vi "AD5781SetVolt.vi"(3 "Send":bool=TRUE, 5 "SetVolt":u32 format="%032b") -> (2 "timedOut":bool)   [LabVIEW 2014]
uses:
  <vilib>/rvi/Emulation/niFpgaGetClockAttributes.vi
  <vilib>/rvi/Emulation/niFpgaSctlEmulationGetInTimedLoop.vi
  <vilib>/rvi/Emulation/niFpgaEmulationReportErrorSimple.vi
  <vilib>/rvi/Emulation/niFpgaCriticalErrorInLSC.vi
  <vilib>/rvi/interface/RandomDataEmulation/niFpgaRandomDataHandleErrors.vi
  <vilib>/rvi/DataTransferAndStorage/Container/XNode/niFpgaContainer.xnode
  <vilib>/rvi/interface/RandomDataEmulation/nirviRandomDataFpgaReadWriteTemplate.vi
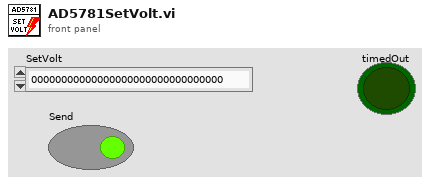
[diagram p1: front panel]
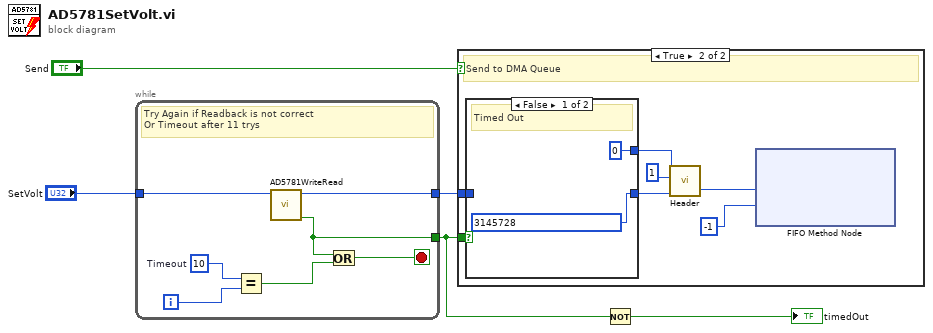
[diagram p0: block diagram]
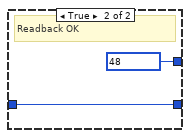
[diagram p3: hidden frame]
diagram:
  n1 = while {
    tunnel: "SetVolt" -> [w12]
    tunnel: [w7] -> w4
    tunnel: [w6] -> w3
    i -> [w11]
    stop <- w9 stop-if-true
    w10 = 10  # Timeout
    # "Try Again if Readback is not correct\nOr Timeout after 11 trys"
    n2 = Equal?(x=w10, y=w11) -> (x = y?=w8:bool)
    n3 = call "AD5781WriteRead.vi"("Write"=w12) -> ("WriteEqualsRead"=w6:bool, "Readback"=w7:u32)  [unwired: 6 in]
    n4 = Or(x=w6, y=w8) -> (x .or. y?=w9:bool)
  }
  n5 = case shown="True" "Send" {
    tunnel: w4 -> [_ w15]
    tunnel: w3 -> [_ w13]
    frame False {
    }
    frame True {
      # "Send to DMA Queue"
      n6 = case shown="False" w13 {
        tunnel: [u8 0 ("8BitHead") u8 48 ("8BitHead")] -> w19
        tunnel: w15 -> [_ w22]
        tunnel: [u32 3145728 ("Readback") w22] -> w14
        frame False {
          # "Timed Out"
        }
        frame True {
          # "Readback OK"
        }
      }
      n7 = call "Header.vi"("23BitData"=w14, "1BitHeaderIndex"=u8 1, "8BitHead"=w19) -> ("32BitOutput"=w17:u32)  [unwired: 2 in]
      n8 = xnode ("FIFO Method Node")("Element"=w17, "Timeout"=-1) -> ()  [unwired: 1 in, 2 out]
    }
  }
  n9 = Not(x=w3) -> (.not. x?=→"timedOut":bool)
